vi "GOOP_DrawProductPicture.vi"(11 "ProductPictureControl":refnum<vi>) -> (3 "Zoom Factor":sgl)   [LabVIEW 2020]
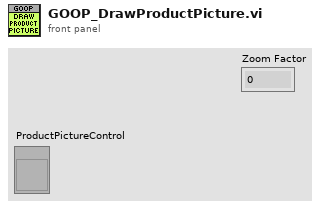
[diagram p1: front panel]
types:
  T1 = typedef "LVBoundsTypeDef.ctl" = cluster{"Width":u32, "Height":u32}
  T2 = typedef "imagedata.ctl" = cluster{"image type":i32, "image depth":i32, "image":u8[], "mask":u8[], "colors":u32[], "Rectangle":cluster{"left":i16, "top":i16, "right":i16, "bottom":i16}}
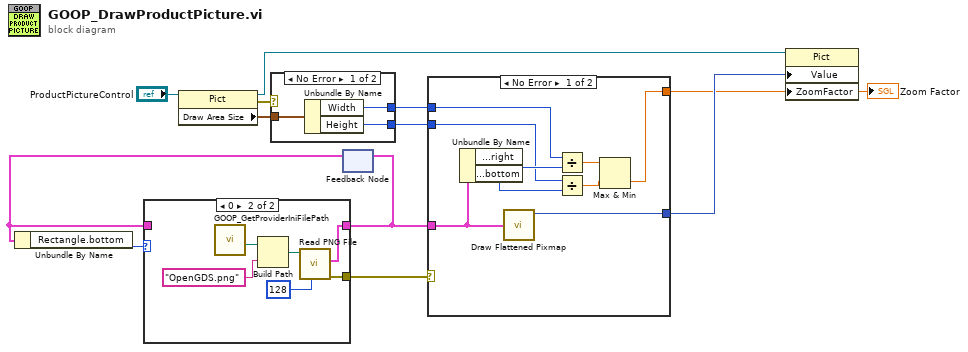
[diagram p0: block diagram]
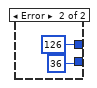
[diagram p2: hidden frame]
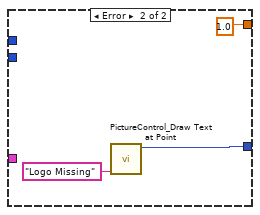
[diagram p3: hidden frame]
diagram:
  n1 = property class="Pict"(reference="ProductPictureControl") -> (reference out=w10:refnum<vi>, error out=w6:errorcluster, "Draw Area Size"=w11:T1)  [unwired: 1 in]
  n2 = case shown="No Error" w6 {
    tunnel: w11 -> [w15 _]
    tunnel: [w14 u32 126 ("Width")] -> w5
    tunnel: [w13 u32 36 ("Height")] -> w4
    frame No Error {
      n3 = Unbundle By Name(w15) -> ("Width"=w14:u32, "Height"=w13:u32)
    }
    frame Error {
    }
  }
  n4 = feedback #1() -> (w9:T2)  [unwired: 1 in]
  n5 = Unbundle By Name(w9) -> ("Rectangle.bottom"=w1:i16)
  n6 = case shown="0" w1 {
    tunnel: [w18 w24] -> w2
    tunnel: w9 -> [w18 _]
    tunnel: [_ w20] -> w8
    frame Default {
    }
    frame 0 {
      n7 = call "GOOP_GetProviderIniFilePath.vi"() -> ("ProviderMainFolder"=w23:path)  [unwired: 10 in, 1 out]
      n8 = Build Path(base path=w23, name or relative path="OpenGDS.png") -> (appended path=w21:path)
      n9 = call <vilib>:"Read PNG File.vi"("Transparency Thresh"=u8 128, "path to PNG file"=w21) -> ("error out"=w20:errorcluster, "image data"=w24:T2)  [unwired: 7 in, 1 out]
    }
  }
  n10 = feedback-in #1(w2) -> ()
  n11 = case shown="No Error" w8 {
    tunnel: w2 -> [w32 _]
    tunnel: [w33 w36] -> w7
    tunnel: w5 -> [w30 _]
    tunnel: w4 -> [w28 _]
    tunnel: [w25 sgl 1.0 ("Zoom Factor")] -> w3
    frame No Error {
      n12 = Unbundle By Name(w32) -> ("Rectangle.right"=w31:i16, "Rectangle.bottom"=w29:i16)
      n13 = call <vilib>:"Draw Flattened Pixmap.vi"("image data"=w32) -> ("new picture"=w33:picture)  [unwired: 8 in]
      n14 = Divide(x=w30, y=w31) -> (x/y=w27:dbl)
      n15 = Divide(x=w28, y=w29) -> (x/y=w26:dbl)
      n16 = Max & Min(x=w27, y=w26) -> (min(x,y)=w25:dbl)  [unwired: 1 out]
    }
    frame Error {
      n17 = call "PictureControl_Draw Text at Point.vi"("text"="Logo Missing") -> ("new picture"=w36:picture)  [unwired: 9 in, 1 out]
    }
  }
  "Zoom Factor" <- w3
  n18 = property class="Pict"(reference=w10, "Value"=w7, "ZoomFactor"=w3) -> ()  [unwired: 1 in, 2 out]
